vi "Read WPROT.vi"(8 "error in (no error)":errorcluster, 11 "Instrument in":refnum<class "Instrument.lvclass">) -> (0 "error out":errorcluster, 2 "Opt_Selector.lvclass":refnum<class "Opt_Selector.lvclass">, 3 "Instrument out":refnum<class "Instrument.lvclass">)   [LabVIEW 2018, in "Instrument.lvclass"]
uses:
  Instrument.lvclass
  Device/Optics/Opt_Selector/Opt_Selector.lvclass
  Instrument.lvclass/Instrument.ctl
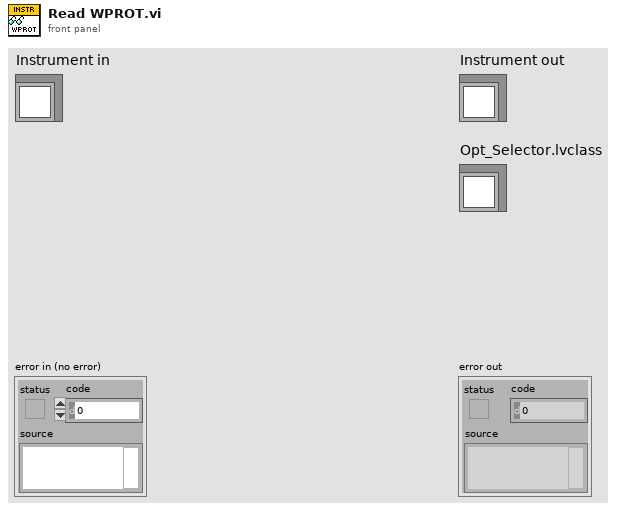
[diagram p1: front panel]
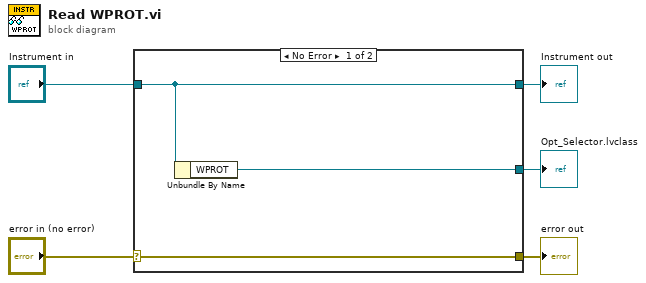
[diagram p0: block diagram]
diagram:
  n1 = case shown="No Error" "error in (no error)" {
    selector: "error in (no error)" -> [w8 w9]
    tunnel: [w8 w9] -> w4
    tunnel: [w7 w10] -> w2
    tunnel: "Instrument in" -> [w7 w10]
    tunnel: [w6 _] -> w1
    frame No Error {
      n2 = Unbundle By Name(w7) -> ("WPROT"=w6:refnum<class "Opt_Selector.lvclass">)
    }
    frame Error {
    }
  }
  "error out" <- w4
  "Instrument out" <- w2
  "Opt_Selector.lvclass" <- w1
